vi "lectura_simultanea_case.vi"(10 "Address Type":T1=1 items=["Public", "Random"], 11 "COM Bluegiga in":refnum<visa-resource-name>="COM13") -> (3 "Connected":bool)   [LabVIEW 2020]
uses:
  <vilib>/BLE/type_def/connection_status_bundle.ctl
  <vilib>/BLE/type_def/address_type.ctl
  <vilib>/Utility/file.llb/Read Delimited Spreadsheet (string).vi
panel:
  out "Humedad":string caption="Result"
  out "UIDS":string[][](array[string])
  out "characteristic value":u8[](array[numeric])
  out "TVOC ppb":u8
  out "eCO2 ppm":u8
  out "Color":u32(colorbox)
  in  "Stop Color":bool
  in  "Quaternion":bool
  out "Presión":dbl
  out "Temp":dbl
  out "Temperatura":string caption="Result"
  out "z 4":dbl
  out "y 4":dbl
  out "x 4":dbl
  out "w 4":dbl
  in  "stop":bool
  out "MAC Address":string
  out "Handle table":string[][](array[string])
  out "Connection Status":T2={"MAC Address"="", "cnx handle"=0, "cnx flags"=0, "Address Type"=125, "Connection Interval (ms)"=125, "Timeout(ms)"=125, "Latency"=0, "bonding handle"=0} {"Address Type" items=["Public", "Random"]}
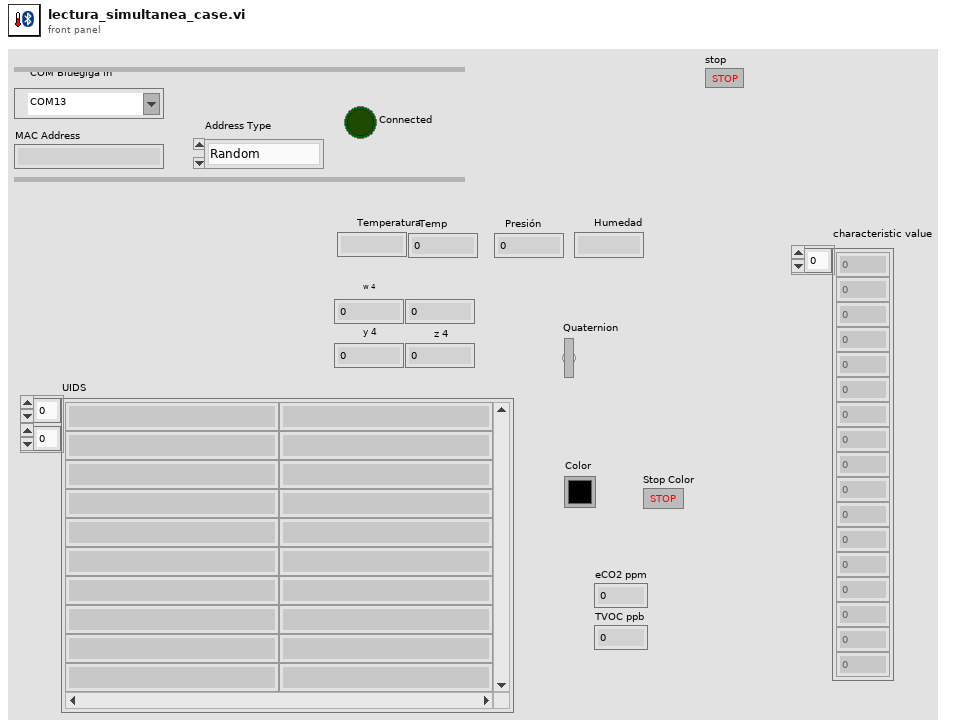
[diagram p1: front panel]
types:
  T1 = typedef "address_type.ctl" = u8
  T2 = typedef "connection_status_bundle.ctl" = cluster{"MAC Address":string, "cnx handle":u8, "cnx flags":u8, "Address Type":T1, "Connection Interval (ms)":u16, "Timeout(ms)":u16, "Latency":u16, "bonding handle":u8}
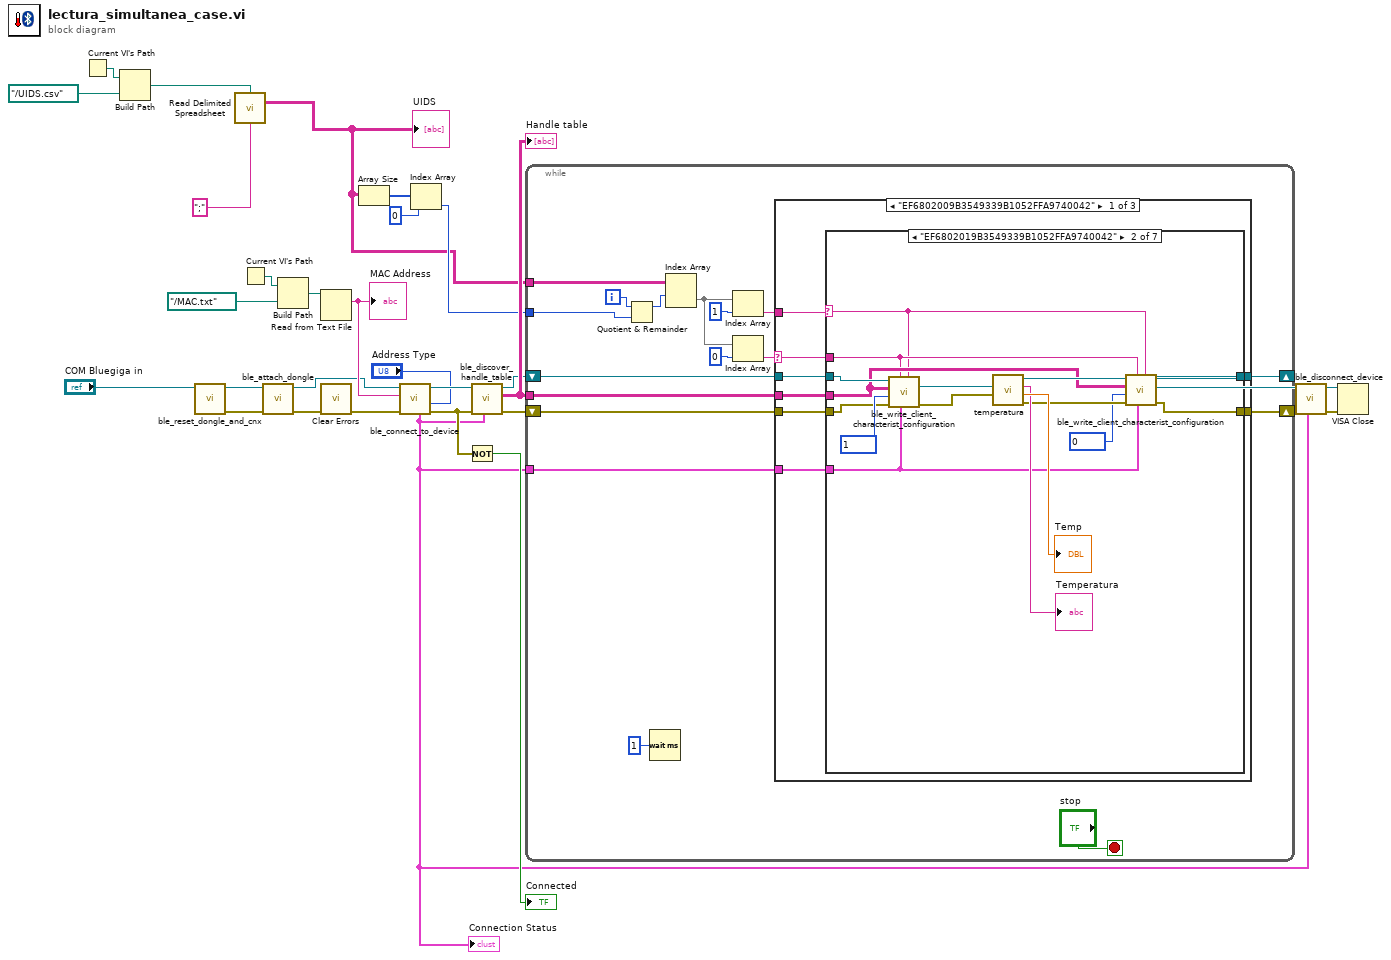
[diagram p0: block diagram]
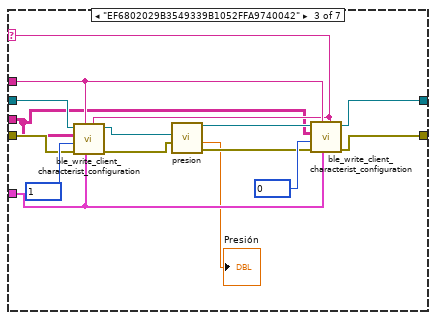
[diagram p3: hidden frame]
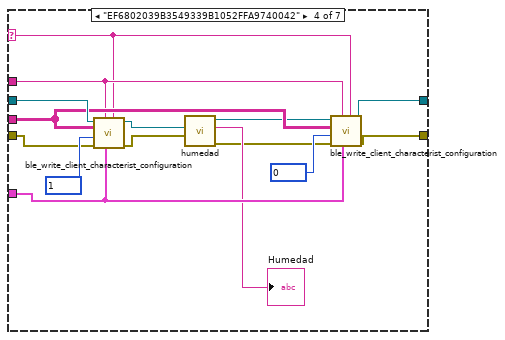
[diagram p4: hidden frame]
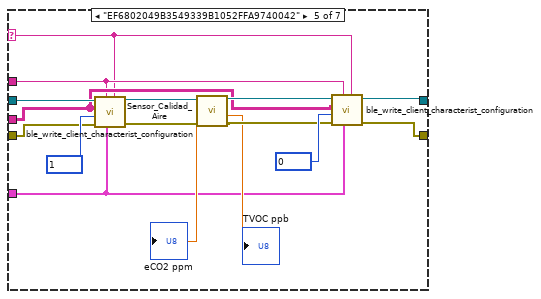
[diagram p5: hidden frame]
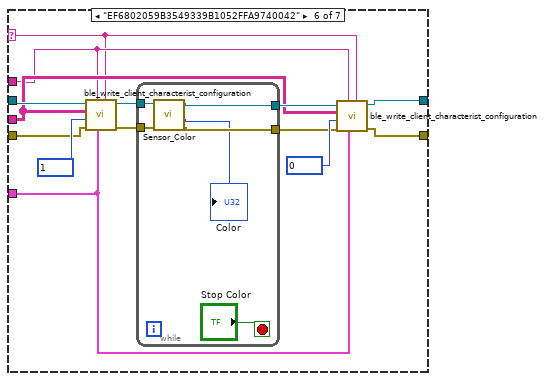
[diagram p6: hidden frame]
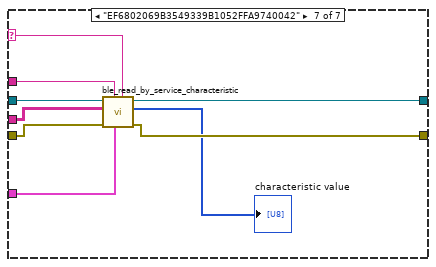
[diagram p7: hidden frame]
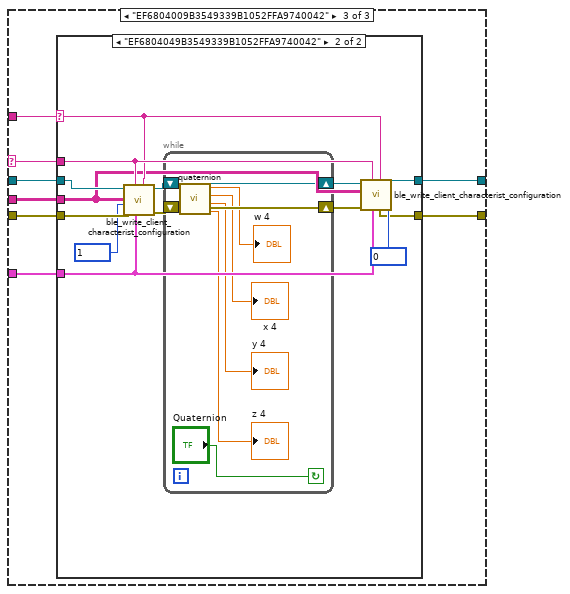
[diagram p9: hidden frame]
diagram:
  n1 = Current VI's Path() -> (path=w7:path)
  n2 = Build Path(base path=w7, name or relative path=path "../UIDS.csv") -> (appended path=w6:path)
  n3 = call <vilib>:"ble_reset_dongle_and_cnx.vi"("COM Bluegiga in"="COM Bluegiga in") -> ("error out"=w28:errorcluster, "COM Bluegiga out"=w26:refnum<visa-resource-name>)  [unwired: 9 in]
  n4 = call-poly <vilib>:"Read Delimited Spreadsheet.vi"("file path (dialog if empty)"=w6, "delimiter (\\t)"=";" ("delimiter (\\t)")) -> ("all rows"=w2:string[][])  [unwired: 8 in, 5 out]
  "UIDS" <- w2
  n5 = Current VI's Path() -> (path=w18:path)
  n6 = call <vilib>:"ble_attach_dongle.vi"("error in (no error)"=w28, "COM Bluegiga in"=w26) -> ("error out"=w16:errorcluster, "COM Bluegiga out"=w17:refnum<visa-resource-name>)  [unwired: 8 in]
  n7 = Build Path(base path=w18, name or relative path=path "../MAC.txt") -> (appended path=w19:path)
  n8 = Read from Text File(file (use dialog)=w19) -> (text=w21:string)  [unwired: 3 in, 3 out]
  "MAC Address" <- w21
  n9 = call <vilib>:"Clear Errors.vi"("error in (no error)"=w16) -> ("error out"=w23:errorcluster)  [unwired: 5 in, 1 out]
  n10 = Array Size(array=w2) -> (size(s)=w4:i32[])
  n11 = call <vilib>:"ble_connect_to_device.vi"("Address Type"="Address Type", "error in (no error)"=w23, "MAC Address"=w21, "COM Bluegiga in"=w17) -> ("error out"=w24:errorcluster, "COM Bluegiga out"=w25:refnum<visa-resource-name>, "Connection Status"=w12:T2)  [unwired: 5 in]
  "Connection Status" <- w12
  n12 = Index Array(array=w4, index=0) -> (element=w3:i32)
  n13 = Not(x=w24) -> (.not. x?=→"Connected":bool)
  n14 = call <vilib>:"ble_discover_handle_table.vi"("Connection Status"=w12, "error in (no error)"=w24, "COM Bluegiga in"=w25) -> ("error out"=w10:errorcluster, "Handle table"=w11:string[][], "COM Bluegiga out"=w9:refnum<visa-resource-name>)  [unwired: 6 in]
  "Handle table" <- w11
  n15 = while {
    tunnel: w2 -> [w32]
    shift-right: [w44] -> w13
    shift-left: w10 -> [w47]
    shift-right: [w45] -> w14
    shift-left: w9 -> [w46]
    tunnel: w12 -> [w43]
    tunnel: w11 -> [w42]
    tunnel: w3 -> [w31]
    i -> [w41]
    stop <- "stop" stop-if-true
    n16 = Quotient & Remainder(x=w41, y=w31) -> (x-y*floor(x/y)=w39:i32)  [unwired: 1 out]
    n17 = Wait (ms)(milliseconds to wait=u32 1) -> ()  [unwired: 1 out]
    n18 = Index Array(array=w32, index (row)=w39) -> (element=w38:string[])  [unwired: 1 in]
    n19 = Index Array(array=w38, index=1) -> (element=w34:string)
    n20 = Index Array(array=w38, index=0) -> (element=w35:string)
    n21 = case shown="\"EF6802009B3549339B1052FFA9740042\"" w35 {
      selector: w35 -> [w54 _ w151]
      tunnel: w47 -> [w51 w149 w156]
      tunnel: w46 -> [w53 w150 w157]
      tunnel: [w49 w150 w154] -> w45
      tunnel: [w48 w149 w153] -> w44
      tunnel: w43 -> [w50 _ w155]
      tunnel: w42 -> [w52 _ w152]
      tunnel: w34 -> [w55 _ w158]
      frame "EF6802009B3549339B1052FFA9740042" {
        n22 = case shown="\"EF6802019B3549339B1052FFA9740042\"" w55 {
          selector: w55 -> [_ w58 w80 w98 w107 w121 w142]
          tunnel: w54 -> [_ w59 w81 w99 w108 w122 w141]
          tunnel: w53 -> [w57 w65 w79 w102 w113 w125 w148]
          tunnel: w52 -> [_ w63 w77 w100 w109 w123 w147]
          tunnel: w51 -> [w56 w64 w78 w101 w110 w124 w146]
          tunnel: w50 -> [_ w62 w84 w97 w104 w120 w145]
          tunnel: [w57 w60 w75 w96 w112 w127 w143] -> w49
          tunnel: [w56 w61 w74 w95 w111 w126 w144] -> w48
          frame Default {
          }
          frame "EF6802019B3549339B1052FFA9740042" {
            n23 = call <vilib>:"ble_write_client_characterist_configuration.vi"("Characteristic UUID"=w58, "Connection Status"=w62, "Service UUID"=w59, "error in (no error)"=w64, "Value(16bit)"=u16 1, "Handle table"=w63, "COM Bluegiga in"=w65) -> ("error out"=w71:errorcluster, "COM Bluegiga out"=w70:refnum<visa-resource-name>)  [unwired: 3 in]
            n24 = call "temperatura.vi"("error in (no error)"=w71, "COM Bluegiga in"=w70) -> ("error out"=w69:errorcluster, "Numeric"=→"Temp":dbl, "Text"=→"Temperatura":string, "COM Bluegiga out"=w68:refnum<visa-resource-name>)  [unwired: 6 in]
            n25 = call <vilib>:"ble_write_client_characterist_configuration.vi"("Characteristic UUID"=w58, "Connection Status"=w62, "Service UUID"=w59, "error in (no error)"=w69, "Value(16bit)"=u16 0, "Handle table"=w63, "COM Bluegiga in"=w68) -> ("error out"=w61:errorcluster, "COM Bluegiga out"=w60:refnum<visa-resource-name>)  [unwired: 3 in]
          }
          frame "EF6802029B3549339B1052FFA9740042" {
            n26 = call <vilib>:"ble_write_client_characterist_configuration.vi"("Characteristic UUID"=w80, "Connection Status"=w84, "Service UUID"=w81, "error in (no error)"=w78, "Value(16bit)"=u16 1, "Handle table"=w77, "COM Bluegiga in"=w79) -> ("error out"=w85:errorcluster, "COM Bluegiga out"=w86:refnum<visa-resource-name>)  [unwired: 3 in]
            n27 = call "presion.vi"("error in (no error)"=w85, "COM Bluegiga in"=w86) -> ("error out"=w83:errorcluster, "Presión"=→"Presión":dbl, "COM Bluegiga out"=w82:refnum<visa-resource-name>)  [unwired: 7 in]
            n28 = call <vilib>:"ble_write_client_characterist_configuration.vi"("Characteristic UUID"=w80, "Connection Status"=w84, "Service UUID"=w81, "error in (no error)"=w83, "Value(16bit)"=u16 0, "Handle table"=w77, "COM Bluegiga in"=w82) -> ("error out"=w74:errorcluster, "COM Bluegiga out"=w75:refnum<visa-resource-name>)  [unwired: 3 in]
          }
          frame "EF6802039B3549339B1052FFA9740042" {
            n29 = call <vilib>:"ble_write_client_characterist_configuration.vi"("Characteristic UUID"=w98, "Connection Status"=w97, "Service UUID"=w99, "error in (no error)"=w101, "Value(16bit)"=u16 1, "Handle table"=w100, "COM Bluegiga in"=w102) -> ("error out"=w91:errorcluster, "COM Bluegiga out"=w92:refnum<visa-resource-name>)  [unwired: 3 in]
            n30 = call "humedad.vi"("error in (no error)"=w91, "COM Bluegiga in"=w92) -> ("error out"=w89:errorcluster, "Text"=→"Humedad":string, "COM Bluegiga out"=w90:refnum<visa-resource-name>)  [unwired: 7 in]
            n31 = call <vilib>:"ble_write_client_characterist_configuration.vi"("Characteristic UUID"=w98, "Connection Status"=w97, "Service UUID"=w99, "error in (no error)"=w89, "Value(16bit)"=u16 0, "Handle table"=w100, "COM Bluegiga in"=w90) -> ("error out"=w95:errorcluster, "COM Bluegiga out"=w96:refnum<visa-resource-name>)  [unwired: 3 in]
          }
          frame "EF6802049B3549339B1052FFA9740042" {
            n32 = call <vilib>:"ble_write_client_characterist_configuration.vi"("Characteristic UUID"=w107, "Connection Status"=w104, "Service UUID"=w108, "error in (no error)"=w110, "Value(16bit)"=u16 1, "Handle table"=w109, "COM Bluegiga in"=w113) -> ("error out"=w115:errorcluster, "COM Bluegiga out"=w116:refnum<visa-resource-name>)  [unwired: 3 in]
            n33 = call "Sensor_Calidad_Aire.vi"("COM Bluegiga in"=w116, "error in (no error)"=w115) -> ("COM Bluegiga out"=w117:refnum<visa-resource-name>, "eCO2 ppm"=→"eCO2 ppm":dbl, "TVOC ppb"=→"TVOC ppb":dbl, "error out"=w114:errorcluster)  [unwired: 5 in]
            n34 = call <vilib>:"ble_write_client_characterist_configuration.vi"("Characteristic UUID"=w107, "Connection Status"=w104, "Service UUID"=w108, "error in (no error)"=w114, "Value(16bit)"=u16 0, "Handle table"=w109, "COM Bluegiga in"=w117) -> ("error out"=w111:errorcluster, "COM Bluegiga out"=w112:refnum<visa-resource-name>)  [unwired: 3 in]
          }
          frame "EF6802059B3549339B1052FFA9740042" {
            n35 = call <vilib>:"ble_write_client_characterist_configuration.vi"("Characteristic UUID"=w121, "Connection Status"=w120, "Service UUID"=w122, "error in (no error)"=w124, "Value(16bit)"=u16 1, "Handle table"=w123, "COM Bluegiga in"=w125) -> ("error out"=w130:errorcluster, "COM Bluegiga out"=w131:refnum<visa-resource-name>)  [unwired: 3 in]
            n36 = while {
              tunnel: w131 -> [w137]
              tunnel: w130 -> [w138]
              tunnel: [w136] -> w129
              tunnel: [w135] -> w128
              stop <- "Stop Color" stop-if-true
              n37 = call "Sensor_Color.vi"("COM Bluegiga in"=w137, "error in (no error)"=w138) -> ("COM Bluegiga out"=w136:refnum<visa-resource-name>, "Color"=→"Color":u32, "error out"=w135:errorcluster)  [unwired: 5 in, 1 out]
            }
            n38 = call <vilib>:"ble_write_client_characterist_configuration.vi"("Characteristic UUID"=w121, "Connection Status"=w120, "Service UUID"=w122, "error in (no error)"=w128, "Value(16bit)"=u16 0, "Handle table"=w123, "COM Bluegiga in"=w129) -> ("error out"=w126:errorcluster, "COM Bluegiga out"=w127:refnum<visa-resource-name>)  [unwired: 3 in]
          }
          frame "EF6802069B3549339B1052FFA9740042" {
            n39 = call <vilib>:"ble_read_by_service_characteristic.vi"("Characteristic UUID"=w142, "Connection Status"=w145, "Service UUID"=w141, "error in (no error)"=w146, "Handle table"=w147, "COM Bluegiga in"=w148) -> ("error out"=w144:errorcluster, "characteristic value"=→"characteristic value":u8[], "COM Bluegiga out"=w143:refnum<visa-resource-name>)  [unwired: 3 in]
          }
        }
      }
      frame Default {
      }
      frame "EF6804009B3549339B1052FFA9740042" {
        n40 = case shown="\"EF6804049B3549339B1052FFA9740042\"" w158 {
          selector: w158 -> [_ w165]
          tunnel: w157 -> [w160 w168]
          tunnel: w156 -> [w159 w169]
          tunnel: w155 -> [_ w163]
          tunnel: [w160 w162] -> w154
          tunnel: [w159 w161] -> w153
          tunnel: w152 -> [_ w164]
          tunnel: w151 -> [_ w166]
          frame Default {
          }
          frame "EF6804049B3549339B1052FFA9740042" {
            n41 = call <vilib>:"ble_write_client_characterist_configuration.vi"("Characteristic UUID"=w165, "Connection Status"=w163, "Service UUID"=w166, "error in (no error)"=w169, "Value(16bit)"=u16 1, "Handle table"=w164, "COM Bluegiga in"=w168) -> ("error out"=w172:errorcluster, "COM Bluegiga out"=w171:refnum<visa-resource-name>)  [unwired: 3 in]
            n42 = while {
              shift-right: [w183] -> w174
              shift-left: w172 -> [w181]
              shift-right: [w182] -> w173
              shift-left: w171 -> [w180]
              stop <- "Quaternion" continue-if-true
              n43 = call "quaternion.vi"("error in (no error)"=w181, "COM Bluegiga in"=w180) -> ("z"=→"z 4":dbl, "y"=→"y 4":dbl, "x"=→"x 4":dbl, "w"=→"w 4":dbl, "COM Bluegiga out"=w182:refnum<visa-resource-name>, "error out"=w183:errorcluster)  [unwired: 4 in]
            }
            n44 = call <vilib>:"ble_write_client_characterist_configuration.vi"("Characteristic UUID"=w165, "Connection Status"=w163, "Service UUID"=w166, "error in (no error)"=w174, "Value(16bit)"=u16 0, "Handle table"=w164, "COM Bluegiga in"=w173) -> ("error out"=w161:errorcluster, "COM Bluegiga out"=w162:refnum<visa-resource-name>)  [unwired: 3 in]
          }
        }
      }
    }
  }
  n45 = call <vilib>:"ble_disconnect_device.vi"("Connection Status"=w12, "error in (no error)"=w13, "COM Bluegiga in"=w14) -> ("error out"=w29:errorcluster, "COM Bluegiga out"=w30:refnum<visa-resource-name>)  [unwired: 7 in]
  n46 = VISA Close(VISA resource name=w30, error in (no error)=w29) -> ()  [unwired: 1 out]
